vi "AVL Auto Time.vi"(11 "State":T1) -> (3 "Non-Auto Time":dbl)   [LabVIEW 2021]
uses:
  Controls/AVL Auto Time.ctl
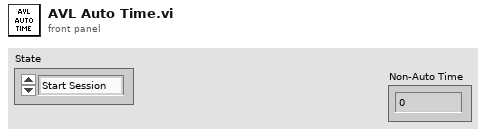
[diagram p1: front panel]
types:
  T1 = typedef "AVL Auto Time.ctl" = enum16{"Start Session", "Exited Auto", "Resumed Auto", "Read Time", "Reload Values"}
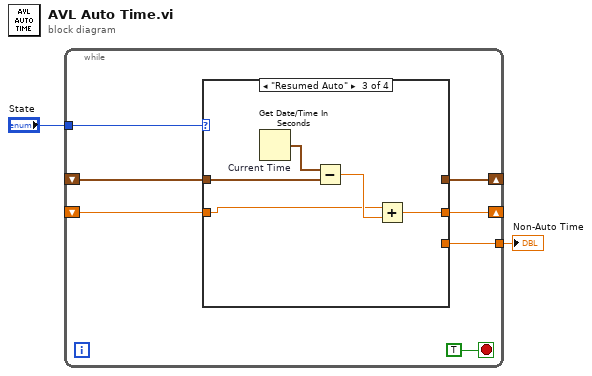
[diagram p0: block diagram]
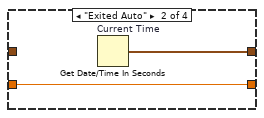
[diagram p3: hidden frame]
diagram:
  n1 = while {
    tunnel: "State" -> [w9]
    shift-right: [w8] -> _
    shift-left: _ -> [w7]
    shift-right: [w6] -> _
    shift-left: _ -> [w5]
    tunnel: [w4] -> w1
    stop <- TRUE stop-if-true
    n2 = case shown="\"Resumed Auto\"" w9 {
      tunnel: [_ w11 _ w18] -> w8
      tunnel: w7 -> [_ _ w14 w18]
      tunnel: [_ w10 w13 w17] -> w6
      tunnel: w5 -> [_ w10 w12 w17]
      tunnel: [_ _ _ w17] -> w4
      frame "Start Session", Default {
      }
      frame "Exited Auto" {
        n3 = Get Date/Time In Seconds "Current Time"() -> (seconds since 1Jan1904=w11:timestamp)
      }
      frame "Resumed Auto" {
        n4 = Get Date/Time In Seconds "Current Time"() -> (seconds since 1Jan1904=w16:timestamp)
        n5 = Subtract(x=w16, y=w14) -> (x-y=w15:dbl)
        n6 = Add(x=w12, y=w15) -> (x+y=w13:dbl)
      }
      frame "Read Time" {
      }
    }
  }
  "Non-Auto Time" <- w1
